vi "ReadExEventFINAL.vi"() -> ()   [LabVIEW 2015]
uses:
  GPS_Driver_Global.vi
panel:
  in  "Path to FITS Header File":path=path "C:/Users/Public/Documents/SI Image SGL II -/Other Parameters.txt"
  out "# Entries After":i16
  in  "# Entries Before":i16
  out "Close Min":u32
  out "Close Maj":u32
  out "Open Min":u32
  out "Open Maj":u32
  out "error out":errorcluster
  in  "error in (no error)":errorcluster
  # "Major UNIX Time:"
  # "Minor UNIX Time:"
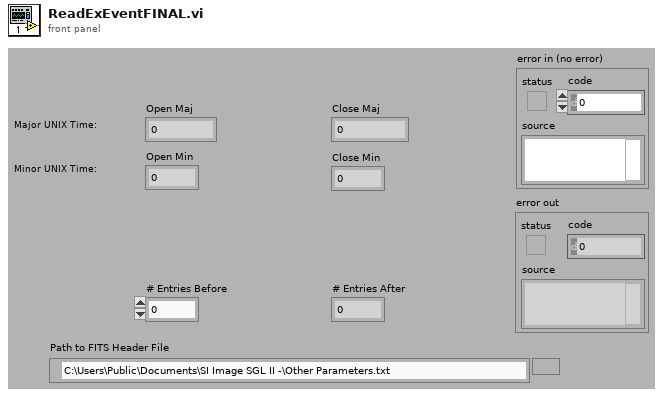
[diagram p1: front panel]
types:
  T1 = cluster{"Close":cluster{"Time":string, "Error":string}, "Open":cluster{"Time":string, "Error":string}, "Date":cluster{"Date":string, "Error":string}}
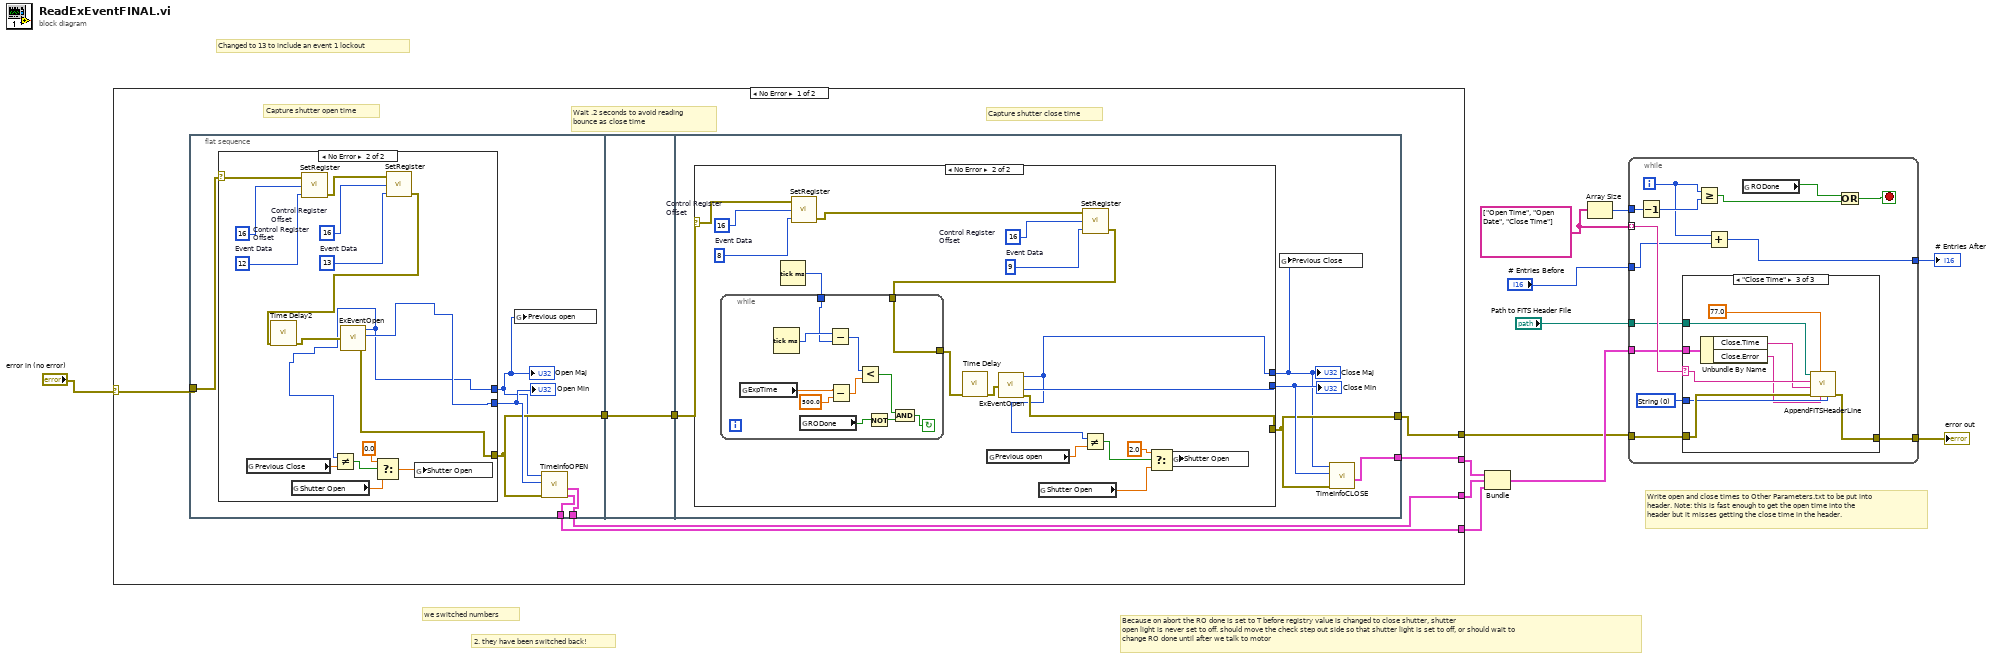
[diagram p0: block diagram]
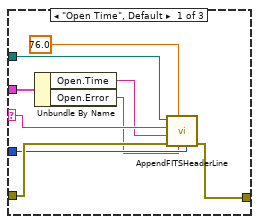
[diagram p2: hidden frame]
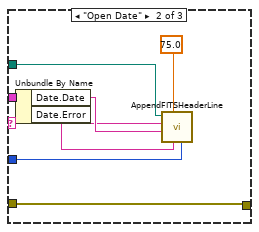
[diagram p3: hidden frame]
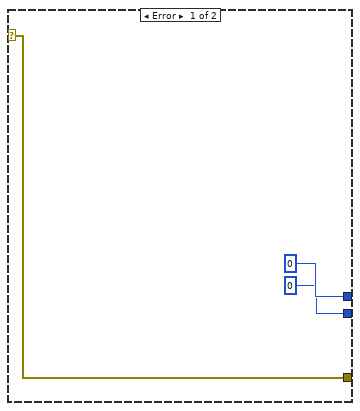
[diagram p4: hidden frame]
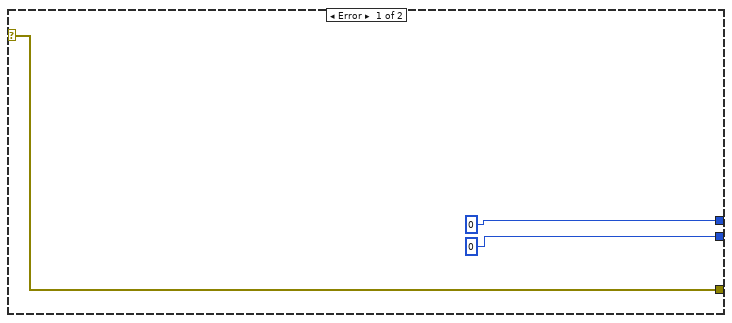
[diagram p5: hidden frame]
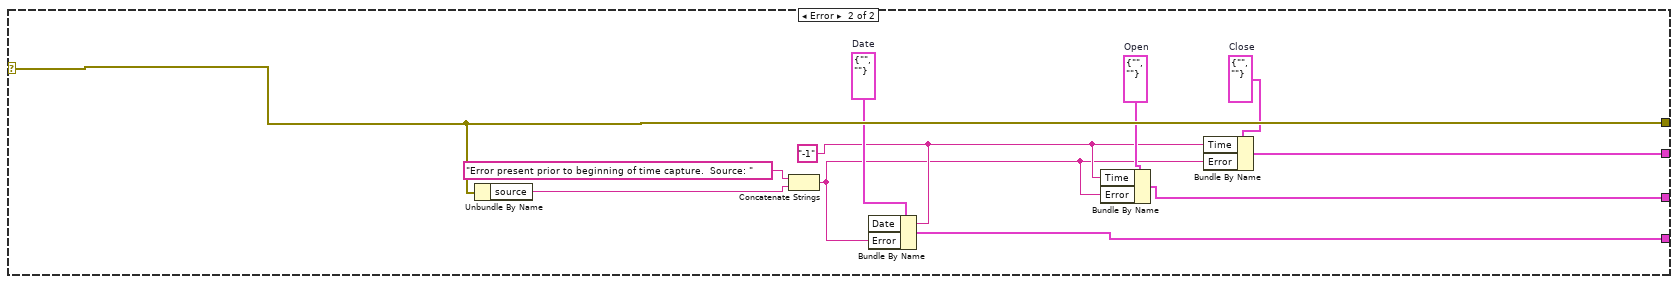
[diagram p6: hidden frame]
diagram:
  w12 = string[] ["Open Time", "Open Date", "Close Time"]
  # "Changed to 13 to include an event 1 lockout"
  # "Because on abort the RO done is set to T before registry value is changed to close shutter, shutter\nopen light is never set to off. should move the check step out side so that shutter light is set to off, or should wait to \nchange RO done until after we talk to motor"
  # "2. they have been switched back!"
  # "we switched numbers"
  # "Write open and close times to Other Parameters.txt to be put into\nheader. Note: this is fast enough to get the open time into the \nheader but it misses getting the close time in the header."
  n1 = case shown="No Error" "error in (no error)" {
    selector: "error in (no error)" -> [w14 w93]
    tunnel: [w13 w93] -> w7
    tunnel: [w19 w86] -> w8
    tunnel: [w18 w89] -> w9
    tunnel: [w15 w87] -> w1
    frame No Error {
      # "Capture shutter close time"
      # "Wait .2 seconds to avoid reading \nbounce as close time"
      # "Capture shutter open time"
      n2 = flat-sequence {
        tunnel: w14 -> [w24]
        tunnel: [w23] -> w19
        tunnel: [w22] -> w16
        tunnel: [w21] -> w15
        tunnel: [w45] -> w17
        tunnel: w16 -> [w45]
        tunnel: [w49] -> w18
        tunnel: w17 -> [w48]
        tunnel: [w47] -> w13
        frame #0 {
          n3 = case shown="No Error" w24 {
            selector: w24 -> [w26 w42]
            tunnel: [0 w39] -> w25
            tunnel: [w26 w41] -> w22
            tunnel: [0 w32] -> w20
            frame Error {
            }
            frame No Error {
              w38 = 13  # Event Data
              w37 = 16  # Control Register Offset
              w43 = 12  # Event Data
              w44 = 16  # Control Register Offset
              n4 = global read "GPS_Driver_Global.vi" "Previous Close"() -> (w33:dbl)
              n5 = global read "GPS_Driver_Global.vi" "Shutter Open"() -> (w29:dbl)
              n6 = call "SetRegister.vi"("Data"=w43, "Offset"=w44, "error in (no error)"=w42) -> ("error out"=w36:errorcluster)  [unwired: 2 in]
              n7 = call "SetRegister.vi"("Data"=w38, "Offset"=w37, "error in (no error)"=w36) -> ("error out"=w35:errorcluster)  [unwired: 2 in]
              n8 = call "Time Delay2"("error in (no error)"=w35) -> ("error out"=w40:errorcluster)  [unwired: 10 in]
              n9 = call "ExEventOpen.vi"("error in (no error)"=w40) -> ("Major Time"=w32:u32, "Minor Time"=w39:u32, "error out"=w41:errorcluster)  [unwired: 1 in]
              n10 = Not Equal?(x=w32, y=w33) -> (x != y?=w31:bool)
              n11 = Select(t=0.0, s=w31, f=w29) -> (s? t:f=w34:dbl)
              n12 = global write "GPS_Driver_Global.vi" "Shutter Open"(w34) -> ()
            }
          }
          "Open Min" <- w25
          "Open Maj" <- w20
          n13 = global write "GPS_Driver_Global.vi" "Previous open"(w20) -> ()
          n14 = call "TimeInfoOPEN.vi"("error in (no error)"=w22, "Minor Time"=w25, "Major Time"=w20) -> ("Date"=w21:cluster{"Date":string, "Error":string}, "Open"=w23:cluster{"Time":string, "Error":string})  [unwired: 6 in]
        }
        frame #1 {
        }
        frame #2 {
          n15 = case shown="No Error" w48 {
            selector: w48 -> [w51 w69]
            tunnel: [0 w67] -> w50
            tunnel: [w51 w68] -> w47
            tunnel: [0 w57] -> w46
            frame Error {
            }
            frame No Error {
              w66 = 9  # Event Data
              w65 = 16  # Control Register Offset
              w70 = 8  # Event Data
              w71 = 16  # Control Register Offset
              n16 = Tick Count (ms)() -> (millisecond timer value=w61:u32)
              n17 = call "SetRegister.vi"("Data"=w70, "Offset"=w71, "error in (no error)"=w69) -> ("error out"=w64:errorcluster)  [unwired: 2 in]
              n18 = global read "GPS_Driver_Global.vi" "Previous open"() -> (w58:dbl)
              n19 = global read "GPS_Driver_Global.vi" "Shutter Open"() -> (w59:dbl)
              n20 = call "SetRegister.vi"("Data"=w66, "Offset"=w65, "error in (no error)"=w64) -> ("error out"=w60:errorcluster)  [unwired: 2 in]
              n21 = while {
                tunnel: w61 -> [w81]
                tunnel: w60 -> [w80]
                tunnel: [w80] -> w55
                stop <- w76 continue-if-true
                n22 = global read "GPS_Driver_Global.vi" "ExpTime"() -> (w74:dbl)
                n23 = Tick Count (ms)() -> (millisecond timer value=w82:u32)
                n24 = global read "GPS_Driver_Global.vi" "RODone"() -> (w79:bool)
                n25 = Subtract(x=w82, y=w81) -> (x-y=w75:u32)
                n26 = Subtract(x=w74, y=500.0) -> (x-y=w73:dbl)
                n27 = Less?(x=w75, y=w73) -> (x < y?=w77:bool)
                n28 = Not(x=w79) -> (.not. x?=w78:bool)
                n29 = And(x=w77, y=w78) -> (x .and. y?=w76:bool)
              }
              n30 = call "Time Delay"("error in (no error)"=w55) -> ("error out"=w54:errorcluster)  [unwired: 10 in]
              n31 = call "ExEventOpen.vi"("error in (no error)"=w54) -> ("Major Time"=w57:u32, "Minor Time"=w67:u32, "error out"=w68:errorcluster)  [unwired: 1 in]
              n32 = Not Equal?(x=w57, y=w58) -> (x != y?=w56:bool)
              n33 = Select(t=2.0, s=w56, f=w59) -> (s? t:f=w62:dbl)
              n34 = global write "GPS_Driver_Global.vi" "Shutter Open"(w62) -> ()
            }
          }
          "Close Maj" <- w46
          "Close Min" <- w50
          n35 = global write "GPS_Driver_Global.vi" "Previous Close"(w46) -> ()
          n36 = call "TimeInfoCLOSE.vi"("error in (no error)"=w47, "Minor Time"=w50, "Major Time"=w46) -> ("Close"=w49:cluster{"Time":string, "Error":string})  [unwired: 7 in]
        }
      }
    }
    frame Error {
      w85 = cluster{"Date":string, "Error":string} {"Date"="", "Error"=""}  # Date
      w90 = cluster{"Time":string, "Error":string} {"Time"="", "Error"=""}  # Close
      w88 = cluster{"Time":string, "Error":string} {"Time"="", "Error"=""}  # Open
      w84 = "-1"
      n37 = Unbundle By Name(w93) -> ("source"=w91:string)
      n38 = Concatenate Strings("Error present prior to beginning of time capture.  Source: ", w91) -> (w83:string)
      n39 = Bundle By Name(cluster=w85, "Date"=w84, "Error"=w83) -> (w87:cluster{"Date":string, "Error":string})
      n40 = Bundle By Name(cluster=w88, "Time"=w84, "Error"=w83) -> (w86:cluster{"Time":string, "Error":string})
      n41 = Bundle By Name(cluster=w90, "Time"=w84, "Error"=w83) -> (w89:cluster{"Time":string, "Error":string})
    }
  }
  n42 = Bundle("Close"=w9, "Open"=w8, "Date"=w1) -> (w11:T1)  [unwired: 1 in]
  n43 = Array Size(array=w12) -> (size(s)=w5:i32)
  n44 = while {
    tunnel: w7 -> [w107]
    tunnel: w12 -> [w105] mode=indexing
    tunnel: w5 -> [w104]
    tunnel: "# Entries Before" -> [w102]
    tunnel: w11 -> [w100]
    tunnel: "Path to FITS Header File" -> [w99]
    tunnel: [w98] -> w10
    tunnel: [w94] -> w3
    i -> [w101]
    stop <- w96 stop-if-true
    w103 = u16 0 items=["String", "Numeric", "Boolean"]
    n45 = Decrement(x=w104) -> (x-1=w106:i32)
    n46 = case shown="\"Close Time\"" w105 {
      selector: w105 -> [w114 w119 w132]
      tunnel: w107 -> [w116 w118 w133]
      tunnel: w103 -> [w115 w123 w131]
      tunnel: w100 -> [w111 w122 w128]
      tunnel: w99 -> [w113 w124 w129]
      tunnel: [w112 w118 w130] -> w98
      frame "Open Time", Default {
        n47 = Unbundle By Name(w111) -> ("Open.Time"=w110:string, "Open.Error"=w109:string)
        n48 = call "AppendFITSHeaderLine.vi"("Entry Type"=w115, "Comment"=w109, "Entry #"=76.0, "error in (no error)"=w116, "Element Value"=w110, "Element Name"=w114, "file path (dialog if empty)"=w113) -> ("error out"=w112:errorcluster)  [unwired: 3 in]
      }
      frame "Open Date" {
        n49 = Unbundle By Name(w122) -> ("Date.Date"=w121:string, "Date.Error"=w120:string)
        n50 = call "AppendFITSHeaderLine.vi"("Entry Type"=w123, "Comment"=w120, "Entry #"=75.0, "Element Value"=w121, "Element Name"=w119, "file path (dialog if empty)"=w124) -> ()  [unwired: 4 in, 1 out]
      }
      frame "Close Time" {
        n51 = Unbundle By Name(w128) -> ("Close.Time"=w127:string, "Close.Error"=w126:string)
        n52 = call "AppendFITSHeaderLine.vi"("Entry Type"=w131, "Comment"=w126, "Entry #"=77.0, "error in (no error)"=w133, "Element Value"=w127, "Element Name"=w132, "file path (dialog if empty)"=w129) -> ("error out"=w130:errorcluster)  [unwired: 3 in]
      }
    }
    n53 = Greater Or Equal?(x=w101, y=w106) -> (x >= y?=w97:bool)
    n54 = Add(x=w101, y=w102) -> (x+y=w94:i32)
    n55 = global read "GPS_Driver_Global.vi" "RODone"() -> (w95:bool)
    n56 = Or(x=w95, y=w97) -> (x .or. y?=w96:bool)
  }
  "error out" <- w10
  "# Entries After" <- w3
